vi "VG-generateFilePath.vi"(8 "file name choises":T1, 9 "Filename":string, 10 "Calibration Folder Path":path, 11 "VG-VNA_GUI in":refnum<class "VG-VNA_GUI.lvclass">) -> (0 "filename out":string="default_calibration_name", 1 "filepath":path, 3 "VG-VNA_GUI out":refnum<class "VG-VNA_GUI.lvclass">)   [LabVIEW 2020, in "VG-VNA_GUI.lvlib" / "VG-VNA_GUI.lvclass"]
uses:
  VG-VNA_GUI.lvclass
  VG-file_name_choices.ctl
  VG-VNA_GUI.lvclass/VG-VNA_GUI.ctl
panel:
  out "resulting string":string
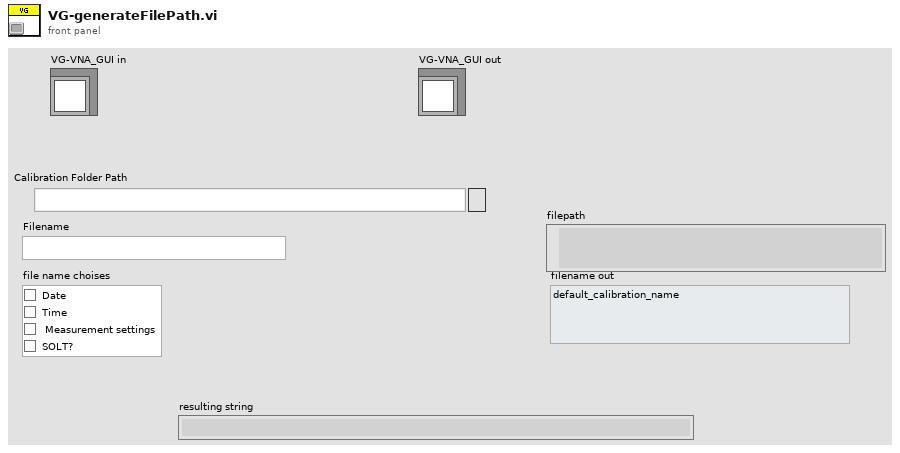
[diagram p1: front panel]
types:
  T1 = typedef "VG-VNA_GUI.lvlib/VG-VNA_GUI.lvclass/VG-file_name_choices.ctl" = cluster{"Date":bool, "Time":bool, "Measurement settings":bool, "SOLT?":bool}
  T2 = typedef "VD-LV-LiteVNA.lvclass/VD-sampleSize.ctl" = u16
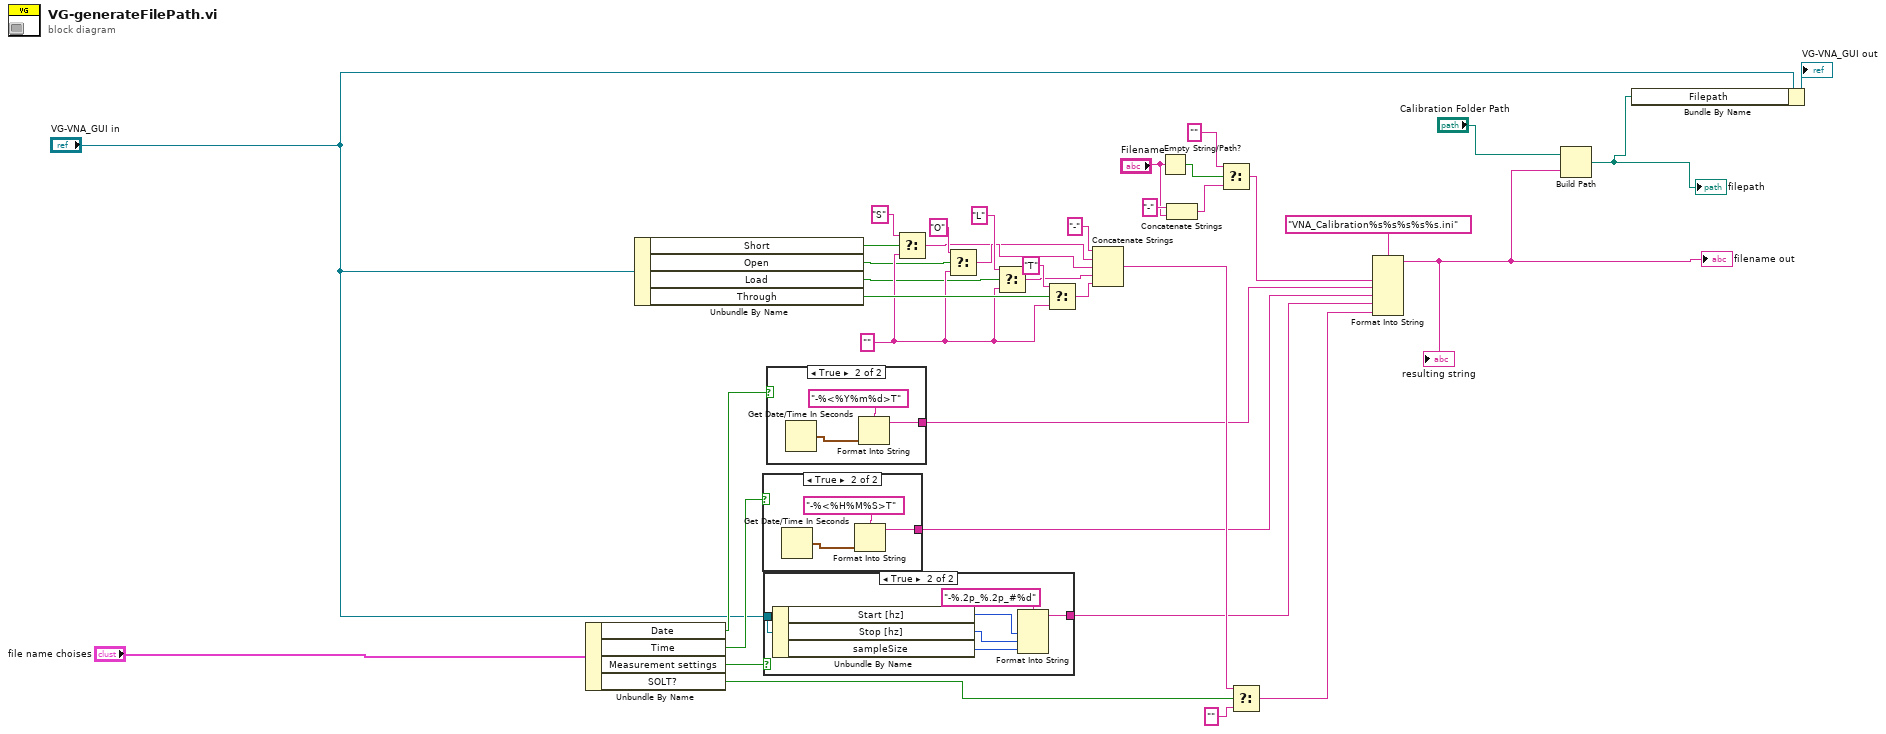
[diagram p0: block diagram]
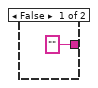
[diagram p2: hidden frame]
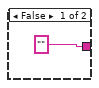
[diagram p3: hidden frame]
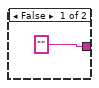
[diagram p4: hidden frame]
diagram:
  w30 = "" ("input 1")
  n1 = Unbundle By Name("file name choises") -> ("Date"=w17:bool, "Time"=w15:bool, "Measurement settings"=w10:bool, "SOLT?"=w34:bool)
  n2 = Unbundle By Name("VG-VNA_GUI in") -> ("Short"=w29:bool, "Open"=w28:bool, "Load"=w27:bool, "Through"=w31:bool)
  n3 = case shown="True" w15 {
    tunnel: ["" w39] -> w14
    frame False {
    }
    frame True {
      n4 = Get Date/Time In Seconds() -> (seconds since 1Jan1904=w40:timestamp)
      n5 = Format Into String(format string="-%<%H%M%S>T", w40) -> (resulting string=w39:string)  [unwired: 2 in, 1 out]
    }
  }
  n6 = case shown="True" w10 {
    tunnel: ["" w48] -> w11
    tunnel: "VG-VNA_GUI in" -> [_ w47]
    frame False {
    }
    frame True {
      n7 = Unbundle By Name(w47) -> ("Start [hz]"=w45:u64, "Stop [hz]"=w44:u64, "sampleSize"=w43:T2)
      n8 = Format Into String(format string="-%.2p_%.2p_#%d", w45, w44, w43) -> (resulting string=w48:string)  [unwired: 2 in, 1 out]
    }
  }
  n9 = case shown="True" w17 {
    tunnel: ["" w50] -> w16
    frame False {
    }
    frame True {
      n10 = Get Date/Time In Seconds() -> (seconds since 1Jan1904=w51:timestamp)
      n11 = Format Into String(format string="-%<%Y%m%d>T", w51) -> (resulting string=w50:string)  [unwired: 2 in, 1 out]
    }
  }
  n12 = Select(t="S", s=w29, f=w30) -> (s? t:f=w19:string)
  n13 = Select(t="O", s=w28, f=w30) -> (s? t:f=w20:string)
  n14 = Select(t="L", s=w27, f=w30) -> (s? t:f=w21:string)
  n15 = Select(t="T", s=w31, f=w30) -> (s? t:f=w22:string)
  n16 = Concatenate Strings("-" ("string"), w19, w20, w21, w22) -> (w18:string)
  n17 = Empty String/Path?(string/path="Filename") -> (empty?=w9:bool)
  n18 = Concatenate Strings("-" ("string"), "Filename") -> (w5:string)
  n19 = Select(t="" ("input 1"), s=w9, f=w5) -> (s? t:f=w4:string)
  n20 = Select(t=w18, s=w34, f="" ("input 1")) -> (s? t:f=w32:string)
  n21 = Format Into String(format string="VNA_Calibration%s%s%s%s%s.ini", w4, w16, w14, w11, w32) -> (resulting string=w3:string)  [unwired: 2 in, 1 out]
  "filename out" <- w3
  "resulting string" <- w3
  n22 = Build Path(base path="Calibration Folder Path", name or relative path=w3) -> (appended path=w1:path)
  "filepath" <- w1
  n23 = Bundle By Name(cluster="VG-VNA_GUI in", "Filepath"=w1) -> (→"VG-VNA_GUI out":refnum<class "VG-VNA_GUI.lvclass">)
